vi "Get Project Path.vi"(11 "Project XML Editor in":refnum<class "Project XML Editor.lvclass">) -> (1 "Available?":bool, 2 "Source Project Path":path, 3 "Project XML Editor out":refnum<class "Project XML Editor.lvclass">)   [LabVIEW 2019, in "LVLIBP CD XML Updater.lvlib" / "Project XML Editor.lvclass"]
uses:
  Project XML Editor.lvclass
  Project XML Editor.lvclass/Project XML Editor.ctl
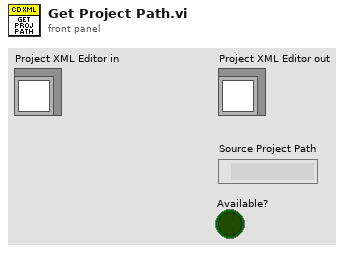
[diagram p1: front panel]
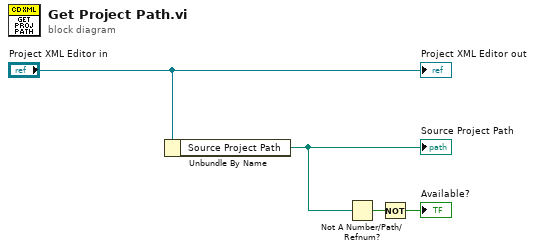
[diagram p0: block diagram]
diagram:
  n1 = Unbundle By Name("Project XML Editor in") -> ("Source Project Path"=w3:path)
  "Source Project Path" <- w3
  n2 = Not A Number/Path/Refnum?(number/path/refnum=w3) -> (NaN/Path/Refnum?=w2:bool)
  n3 = Not(x=w2) -> (.not. x?=→"Available?":bool)
  "Project XML Editor out" <- "Project XML Editor in"
